vi "Contour Plot.vi"() -> ()   [LabVIEW 2011]
uses:
  <vilib>/Heliosphere Research LLC/Advanced Plotting Toolkit/Advanced Plotting Toolkit.lvlib
  <vilib>/Heliosphere Research LLC/Advanced Plotting Toolkit/api_plotting/Contour_Automatic.vi
  <vilib>/Heliosphere Research LLC/Advanced Plotting Toolkit/properties/Line_Style.ctl
  <vilib>/Heliosphere Research LLC/Advanced Plotting Toolkit/typedefs/PlotColor.ctl
  <vilib>/Heliosphere Research LLC/Advanced Plotting Toolkit/properties/Line.ctl
  <vilib>/Heliosphere Research LLC/Advanced Plotting Toolkit/properties/Display.ctl
  <vilib>/Heliosphere Research LLC/Advanced Plotting Toolkit/api_plotting/ContourProperties.ctl
  <vilib>/Heliosphere Research LLC/Advanced Plotting Toolkit/api_plotting/Contour_Manual.vi
panel:
  in  "Auto Contour":bool=TRUE
  in  "Show Labels":bool=TRUE
  in  "Manual Contours":dbl[](array[numeric])=[-0.75, 0.0, 0.125, 1.0]
  in  "Number of Automatic Contours":i32=10
  out "Contour Plot":picture
  # "Contour Plot"
  # "This VI demonstrates how to use contour lines.  Contour lines\nmap out \"levels\" of constant value in a 2D dataset.\n\nProvide a 2D dataset, and specify the levels you would like to\nsee plotted.  Contour.vi is polymorphic; you can either wire\nan integer to the \"Levels\" terminal (automatic contouring),\nor an array of floats specifying the exact levels you would like\nto see.\n\nYou are free to combine Contour.vi with other Toolkit VIs.\nIn this example, the underlying dataset is displayed in false\ncolor using ArrayView.vi.  See also ContourFilled.vi, which\ndisplays filled regions between contours, as opposed to lines."
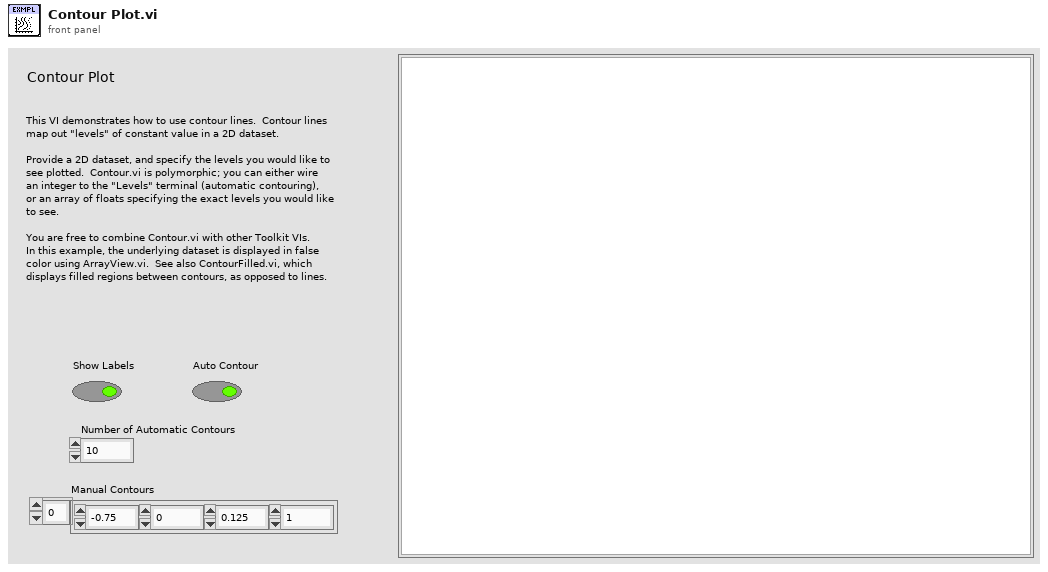
[diagram p1: front panel]
types:
  T1 = typedef "Advanced Plotting Toolkit.lvlib/ContourProperties.ctl" = cluster{"Label Contours":bool, "Line":T2, "Display":T5}
  T2 = typedef "Advanced Plotting Toolkit.lvlib/Line.ctl" = cluster{"Style":T3, "Color":T4, "Width":sgl}
  T3 = typedef "Advanced Plotting Toolkit.lvlib/Line_Style.ctl" = enum16{"Automatic", "Solid", "Dashed", "Dotted", "Dash-dot", "Invisible"}
  T4 = typedef "Advanced Plotting Toolkit.lvlib/PlotColor.ctl" = u32
  T5 = typedef "Advanced Plotting Toolkit.lvlib/Display.ctl" = cluster{"Alpha":dbl, "Z Order":dbl}
  T6 = typedef "Advanced Plotting Toolkit.lvlib/PlotID.ctl" = i32
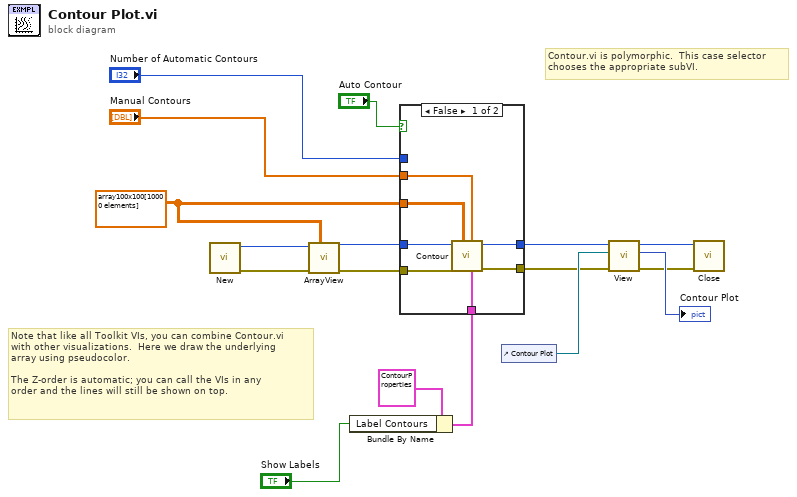
[diagram p0: block diagram]
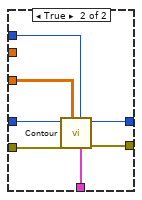
[diagram p2: hidden frame]
diagram:
  w11 = sgl[][] array100x100[10000 elements] ("Array")
  # "Note that like all Toolkit VIs, you can combine Contour.vi\nwith other visualizations.  Here we draw the underlying\narray using pseudocolor.\n\nThe Z-order is automatic; you can call the VIs in any\norder and the lines will still be shown on top."
  # "Contour.vi is polymorphic.  This case selector\nchooses the appropriate subVI."
  n1 = call <vilib>:"New.vi"() -> ("error out"=w4:errorcluster, "Plot ID"=w13:T6)  [unwired: 10 in]
  n2 = call <vilib>:"ArrayView.vi"("Data"=w11, "error in (no error)"=w4, "Plot ID"=w13) -> ("error out"=w3:errorcluster, "Plot ID Out"=w12:T6)  [unwired: 7 in]
  n3 = Bundle By Name(cluster=T1 {"Label Contours"=FALSE, "Line"={"Style"=enum."Automatic", "Color"=2147483647, "Width"=nan}, "Display"={"Alpha"=nan, "Z Order"=nan}} ("Contour Properties"), "Label Contours"="Show Labels") -> (w9:T1)
  n4 = case shown="False" "Auto Contour" {
    tunnel: [w20 w31] -> w14
    tunnel: w12 -> [w21 w30]
    tunnel: w11 -> [w24 w29]
    tunnel: w9 -> [w22 w28]
    tunnel: "Number of Automatic Contours" -> [_ w27]
    tunnel: "Manual Contours" -> [w23 _]
    tunnel: w3 -> [w19 w26]
    tunnel: [w18 w25] -> w2
    frame False {
      n5 = call-poly <vilib>:"Contour.vi"("Properties"=w22, "Levels"=w23, "Z Data"=w24, "error in (no error)"=w19, "Plot ID"=w21) -> ("error out"=w18:errorcluster, "Plot ID Out"=w20:T6)  [unwired: 5 in]
    }
    frame True {
      n6 = call-poly <vilib>:"Contour.vi"("Properties"=w28, "Levels"=w27, "Z Data"=w29, "error in (no error)"=w26, "Plot ID"=w30) -> ("error out"=w25:errorcluster, "Plot ID Out"=w31:T6)  [unwired: 5 in]
    }
  }
  n7 = control-ref of="Contour Plot"() -> (w17:refnum<vi>)
  n8 = call <vilib>:"View.vi"("error in (no error)"=w2, "Ref for Sizing"=w17, "Plot ID"=w14) -> ("error out"=w1:errorcluster, "Picture"=→"Contour Plot":picture, "Plot ID Out"=w15:T6)  [unwired: 6 in]
  n9 = call <vilib>:"Close.vi"("error in (no error)"=w1, "Plot ID"=w15) -> ()  [unwired: 9 in, 1 out]
